vi "Read Input Registers.vi"(8 "error in (no error)":errorcluster, 9 "number of input registers":u16, 10 "starting address":u16, 11 "Modbus master in":refnum<class "Modbus Master.lvclass">) -> (0 "error out":errorcluster, 2 "register values":u16[](array[numeric]), 3 "Modbus master out":refnum<class "Modbus Master.lvclass">)   [LabVIEW 2021, in "Modbus Master.lvclass"]
doc: "Reads values from contiguous input registers. The maximum number of input registers this VI can read is 125."
uses:
  Modbus Master.lvclass
  D:/my_projects/projects/Algorithms/Labview/21/Modbus_v121c/API/Modbus API.lvclass
  Modbus API.lvclass/Modbus API.ctl
  Network Protocol/Network Protocol.lvclass/Network Protocol.ctl
  Modbus Master.lvclass/Modbus Master.ctl
  Transmission Data Unit/Transmission Data Unit.lvclass
  Modbus API.lvclass
  Master Function Definition/Master Function Definition.lvclass
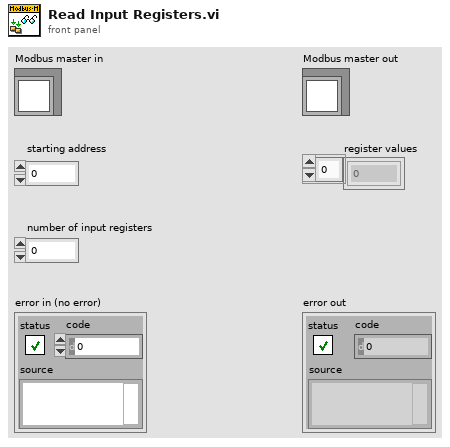
[diagram p1: front panel]
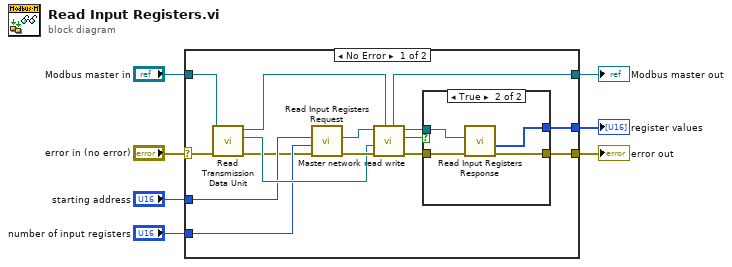
[diagram p0: block diagram]
diagram:
  n1 = case shown="No Error" "error in (no error)" {
    selector: "error in (no error)" -> [w10 w29]
    tunnel: [w20 w29] -> w6
    tunnel: [w15 w28] -> w5
    tunnel: "Modbus master in" -> [w11 w28]
    tunnel: [w16 _] -> w3
    tunnel: "starting address" -> [w14 _]
    tunnel: "number of input registers" -> [w13 _]
    frame No Error {
      n2 = call "Read Transmission Data Unit.vi"("error in"=w10, "Modbus instance in"=w11) -> ("error out"=w8:errorcluster, "transmission data unit"=w17:refnum<class "Transmission Data Unit.lvclass">, "Modbus instance out"=w9:refnum<class "Modbus Master.lvclass">)  [unwired: 7 in]
      n3 = call "Read Input Registers Request.vi"("error in"=w8, "Number of Registers"=w13, "Starting Address"=w14) -> ("error out"=w21:errorcluster, "modbus data unit out"=w18:refnum<class "Modbus Data Unit.lvclass">)  [unwired: 7 in]
      n4 = call "Master network read write.vi"("Modbus master in"=w9, "error in (no error)"=w21, "transmission data unit in"=w17, "Modbus data unit in"=w18) -> ("error out"=w22:errorcluster, "PDU valid?"=w12:bool, "Modbus data unit out"=w19:refnum<class "Modbus Data Unit.lvclass">, "Modbus master out"=w15:refnum<class "Modbus Master.lvclass">)  [unwired: 4 in]
      n5 = case shown="True" w12 {
        tunnel: w22 -> [w23 w27]
        tunnel: [w23 w26] -> w20
        tunnel: w19 -> [_ w25]
        tunnel: [_ w24] -> w16
        frame False {
        }
        frame True {
          n6 = call "Read Input Registers Response.vi"("error in"=w27, "modbus data unit in"=w25) -> ("error out"=w26:errorcluster, "Register Values"=w24:u16[])  [unwired: 7 in, 1 out]
        }
      }
    }
    frame Error {
    }
  }
  "error out" <- w6
  "Modbus master out" <- w5
  "register values" <- w3
